vi "ConvertToRollPitchYaw.vi"(1 "Yaw":bool=TRUE, 2 "Input-Mag":T1, 3 "Input-Gs":T1) -> (0 "Roll Pitch Yaw":T1)   [LabVIEW 2014]
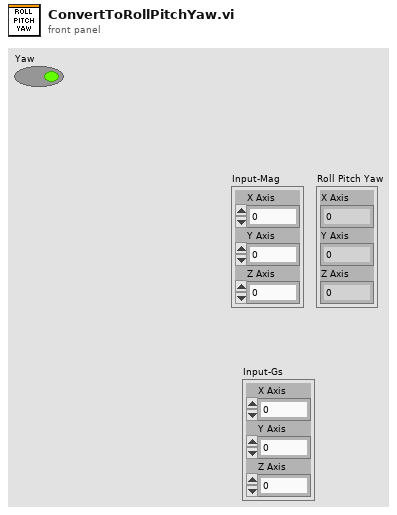
[diagram p1: front panel]
types:
  T1 = cluster{"X Axis":dbl, "Y Axis":dbl, "Z Axis":dbl}
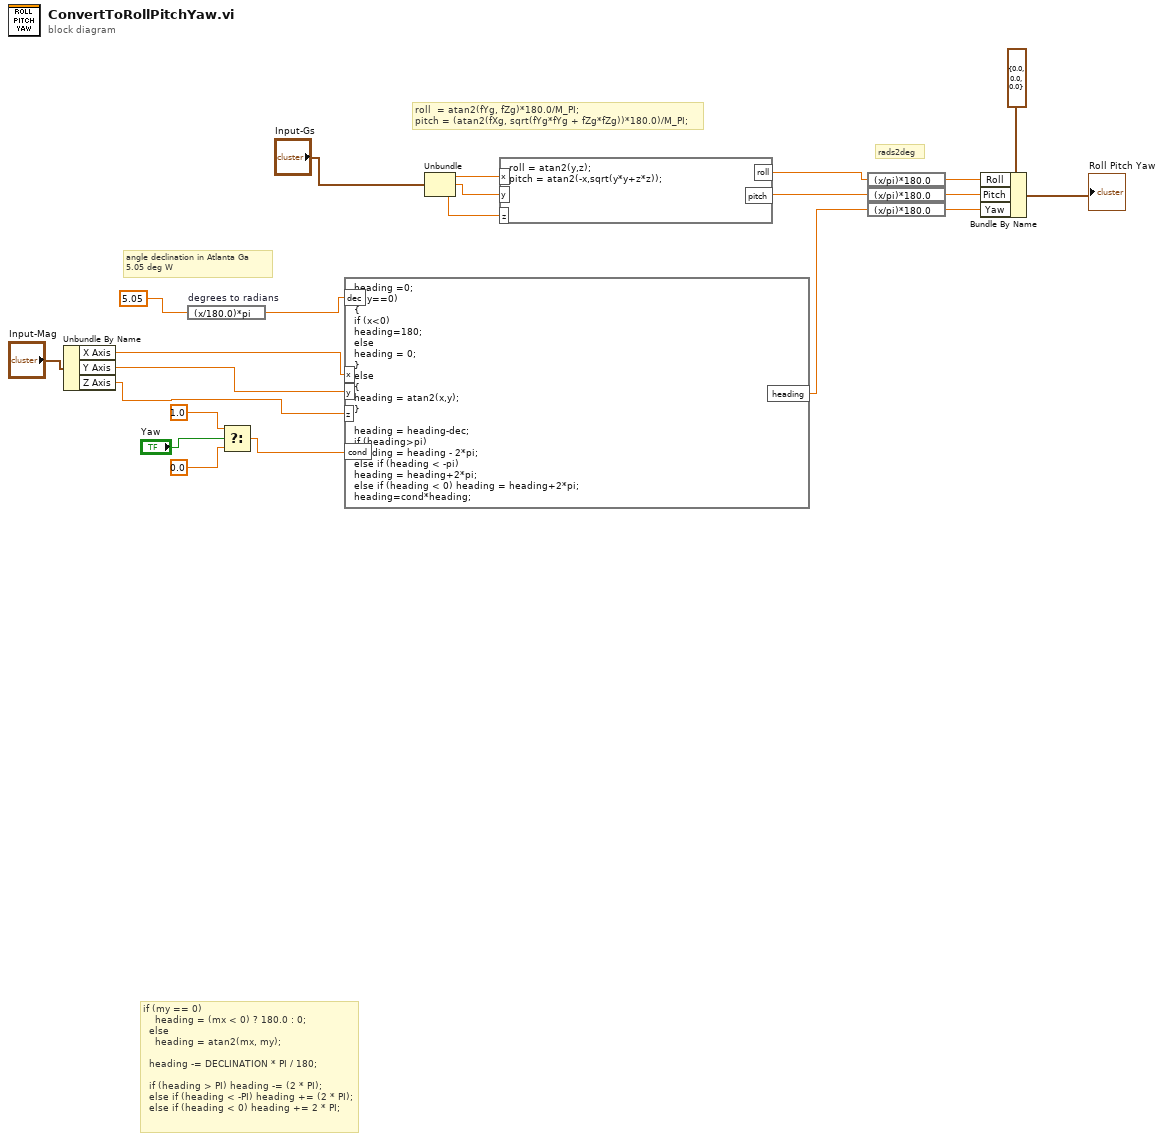
[diagram p0: block diagram]
diagram:
  # "rads2deg"
  # "angle declination in Atlanta Ga\n5.05 deg W"
  # "if (my == 0)\n    heading = (mx < 0) ? 180.0 : 0;\n  else\n    heading = atan2(mx, my);\n    \n  heading -= DECLINATION * PI / 180;\n  \n  if (heading > PI) heading -= (2 * PI);\n  else if (heading < -PI) heading += (2 * PI);\n  else if (heading < 0) heading += 2 * PI;"
  # "roll  = atan2(fYg, fZg)*180.0/M_PI;\npitch = (atan2(fXg, sqrt(fYg*fYg + fZg*fZg))*180.0)/M_PI;"
  n1 = Unbundle By Name("Input-Mag") -> ("X Axis"=w9:dbl, "Y Axis"=w8:dbl, "Z Axis"=w7:dbl)
  n2 = expression code="(x/180.0)*pi" "degrees to radians"(5.05 ("Declination")) -> (w14:dbl)
  n3 = Select(t=1.0, s="Yaw", f=0.0) -> (s? t:f=w10:dbl)
  n4 = formula code="heading =0;\nif (y==0)\n{\nif (x<0)\nheading=180;\nelse\nheading = 0;\n}\nelse\n{\nheading = atan2(x,y);\n}\n\nheading = heading-dec;\nif (heading>pi)\nheading = heading - 2*pi;\nelse if (heading < -pi)\nheading = heading+2*pi;\nelse if (heading < 0) heading = heading+2*pi;\nheading=cond*heading;"("dec"=w14, "cond"=w10, "x"=w9, "y"=w8, "z"=w7) -> ("heading"=w6:dbl)
  n5 = Unbundle("Input-Gs") -> ("X Axis"=w5:dbl, "Y Axis"=w4:dbl, "Z Axis"=w3:dbl)
  n6 = formula code="roll = atan2(y,z);\npitch = atan2(-x,sqrt(y*y+z*z));"("x"=w5, "y"=w4, "z"=w3) -> ("pitch"=w1:dbl, "roll"=w2:dbl)
  n7 = expression code="(x/pi)*180.0" ("radians to degrees")(w2) -> (w21:dbl)
  n8 = expression code="(x/pi)*180.0" ("radians to degrees")(w1) -> (w20:dbl)
  n9 = expression code="(x/pi)*180.0" ("radians to degrees")(w6) -> (w17:dbl)
  n10 = Bundle By Name(cluster=cluster{"Roll":dbl, "Pitch":dbl, "Yaw":dbl} {"Roll"=0.0, "Pitch"=0.0, "Yaw"=0.0} ("input cluster"), "Roll"=w21, "Pitch"=w20, "Yaw"=w17) -> (→"Roll Pitch Yaw":cluster{"Roll":dbl, "Pitch":dbl, "Yaw":dbl})
